vi "write to fifo.vi"(0 "device_type in":refnum<class "device_type.lvclass">, 11 "error in (no error)":errorcluster) -> (4 "device_type out":refnum<class "device_type.lvclass">, 6 "done write file":bool=TRUE, 8 "num of pulses sent to the FPGA":u32, 10 "room on fifo":bool=TRUE, 15 "error out":errorcluster)   [LabVIEW 2021, in "device_type.lvclass"]
uses:
  device_type.lvclass
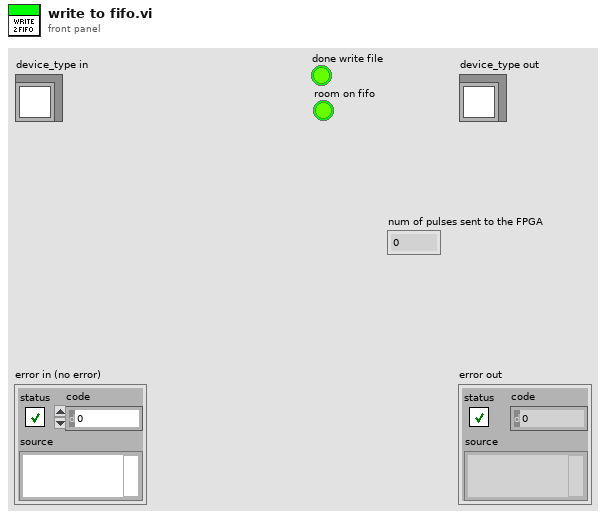
[diagram p1: front panel]
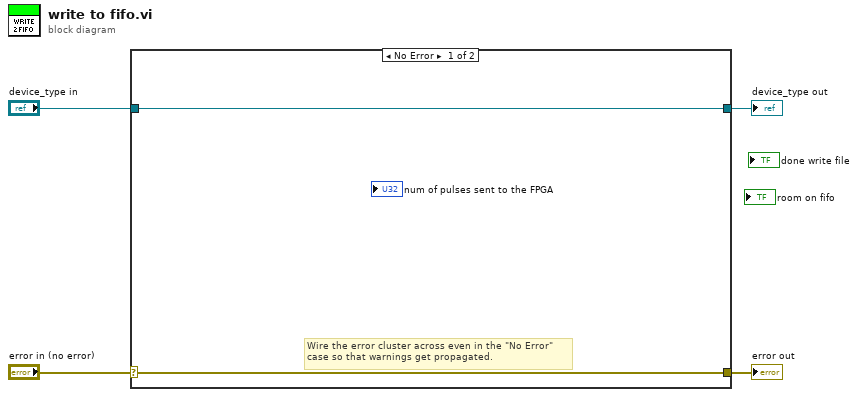
[diagram p0: block diagram]
diagram:
  n1 = case shown="No Error" "error in (no error)" {
    selector: "error in (no error)" -> [w5 w8]
    tunnel: [w5 w8] -> w3
    tunnel: [w6 w7] -> w1
    tunnel: "device_type in" -> [w6 w7]
    frame No Error {
      # "Wire the error cluster across even in the \"No Error\"\ncase so that warnings get propagated."
    }
    frame Error {
    }
  }
  "error out" <- w3
  "device_type out" <- w1
